vi "Launch Process.vi"(8 "error in (no error)":errorcluster, 11 "Service in":refnum<class "Service.lvclass">) -> (0 "error out":errorcluster, 3 "Service out":refnum<class "Service.lvclass">)   [LabVIEW 2024, in "Ramses Framework.lvlib" / "Service.lvclass"]
uses:
  Service.lvclass
  Main Process.vi
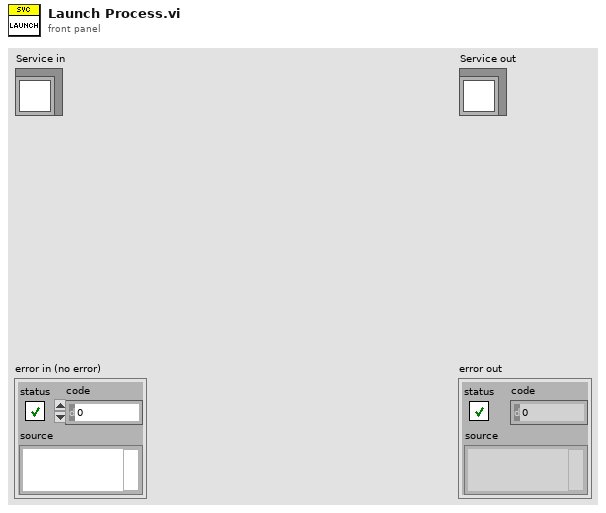
[diagram p1: front panel]
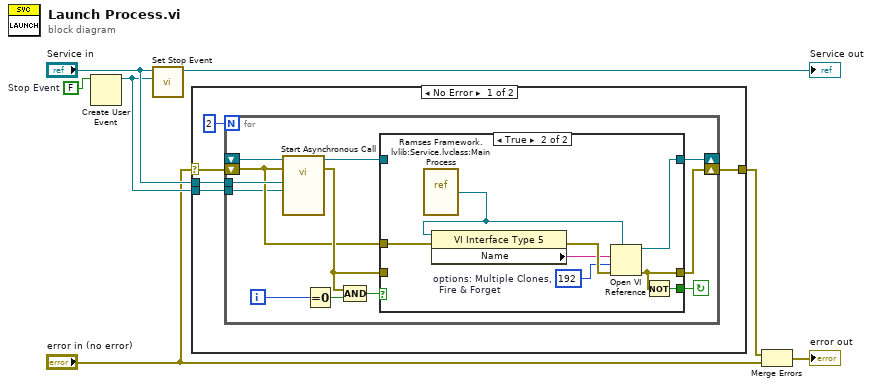
[diagram p0: block diagram]
diagram:
  w5 = FALSE  # Stop Event
  n1 = Create User Event(user event datatype=w5) -> (user event=w2:refnum<user-event>)  [unwired: 1 in, 1 out]
  n2 = call "Set Stop Event.vi"("Stop Event"=w2, "Service in"="Service in") -> ("Service out"=→"Service out":refnum<class "Service.lvclass">)  [unwired: 8 in, 1 out]
  n3 = case shown="No Error" "error in (no error)" {
    selector: "error in (no error)" -> [w9 w35]
    tunnel: "Service in" -> [w12 _]
    tunnel: [w10 w35] -> w7
    tunnel: w2 -> [w8 _]
    frame No Error {
      n4 = for {
        N: 2 -> [_]
        tunnel: w12 -> [w24]
        shift-right: [w23] -> _
        shift-left: _ -> [w22]
        shift-right: [w20] -> w10
        shift-left: w9 -> [w14]
        tunnel: w8 -> [w13]
        i -> [w17]
        stop <- w15 continue-if-true
        n5 = call-by-ref "Start Asynchronous Call"(reference=w22, error in=w14, "Stop Event"=w13, "Service in"=w24) -> (reference out=w21:refnum<vi>, error out=w16:errorcluster)  [unwired: 8 in, 2 out]
        n6 = Equal To 0?(x=w17) -> (x = 0?=w18:bool)
        n7 = Compound Arithmetic op=AND(w16, w18) -> (w19:bool)
        n8 = case shown="True" w19 {
          tunnel: [w26 w31] -> w23
          tunnel: [w25 w29] -> w20
          tunnel: w21 -> [w26 _]
          tunnel: w16 -> [w25 _]
          tunnel: [_ w30] -> w15
          tunnel: w14 -> [_ w28]
          frame False {
          }
          frame True {
            w32 = 192  # options: Multiple Clones,   Fire & Forget
            n9 = vi-ref "Ramses Framework.lvlib:Service.lvclass:Main Process.vi"() -> (w27:refnum<vi>)
            n10 = property class="VI Interface Type 5"(reference=w27, error in=w28) -> (error out=w34:errorcluster, "Name"=w33:string)  [unwired: 1 out]
            n11 = Open VI Reference(type specifier VI Refnum (for type only)=w27, vi path=w33, options=w32, error in (no error)=w34) -> (vi reference=w31:refnum<vi>, error out=w29:errorcluster)  [unwired: 2 in]
            n12 = Not(x=w29) -> (.not. x?=w30:bool)
          }
        }
      }
    }
    frame Error {
    }
  }
  n13 = Merge Errors(w7, "error in (no error)") -> (→"error out":errorcluster)
